vi "Update Generation Signal - Digital.vi"(8 "error in (no error)":errorcluster, 10 "signal update setting":T1, 11 "AudioGeneration in":refnum<class "AudioGeneration.lvclass">) -> (0 "error out":errorcluster, 3 "AudioGeneration out":refnum<class "AudioGeneration.lvclass">)   [LabVIEW 2021, in "AudioGeneration.lvclass"]
uses:
  AudioGeneration.lvclass
  controls/update signal settings.ctl
  <vilib>/NI/STM/TCP/TCP Write Options.ctl
  <vilib>/NI/STM/TCP/Write Message (TCP).vi
  AudioGeneration.lvclass/AudioGeneration.ctl
  <vilib>/NI/STM/NI STM.lvlib
  controls/AudioGenTypeDefs.lvlib
panel:
  out "timeout":bool
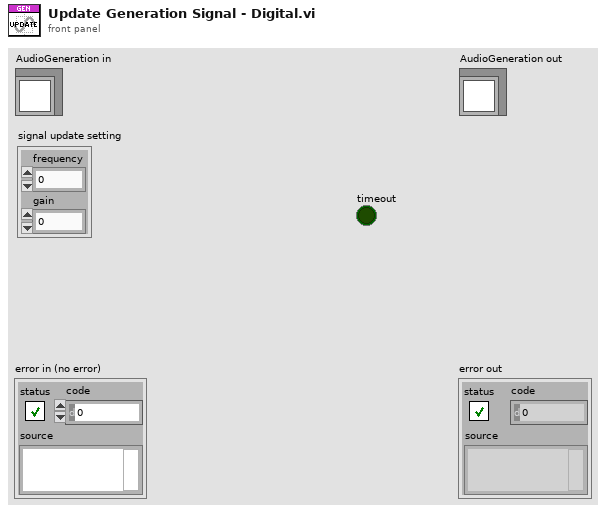
[diagram p1: front panel]
types:
  T1 = typedef "AudioGenTypeDefs.lvlib/update signal settings.ctl" = cluster{"frequency":dbl, "gain":dbl}
  T2 = typedef "NI STM.lvlib/TCP Write Options.ctl" = cluster{"ignore timeout error":bool, "timeout ms (1000)":i32}
  T3 = typedef "NI STM.lvlib/TCP Connection Info.ctl" = cluster{"connection ID":refnum<k5>, "meta data":T4[]}
  T4 = typedef "NI STM.lvlib/MetaDataElement.ctl" = string
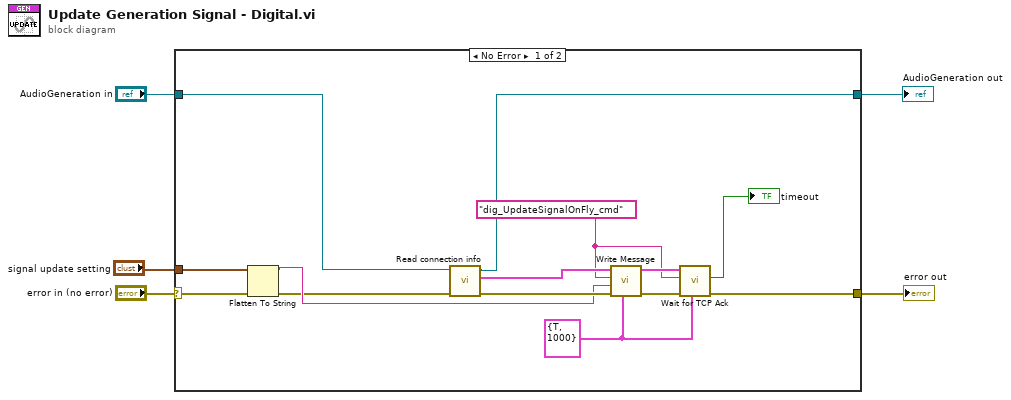
[diagram p0: block diagram]
diagram:
  n1 = case shown="No Error" "error in (no error)" {
    selector: "error in (no error)" -> [w14 w21]
    tunnel: [w16 w21] -> w3
    tunnel: "AudioGeneration in" -> [w7 w20]
    tunnel: [w15 w20] -> w2
    tunnel: "signal update setting" -> [w12 _]
    frame No Error {
      w9 = "dig_UpdateSignalOnFly_cmd" ("name")
      w10 = T2 {"ignore timeout error"=TRUE, "timeout ms (1000)"=1000} ("options")
      n2 = Flatten To String(anything=w12, error in (no error)=w14) -> (data string=w13:string, error out=w6:errorcluster)  [unwired: 2 in, 1 out]
      n3 = call-dynamic "Read connection info.vi"("error in (no error)"=w6, "AudioGeneration in"=w7) -> ("error out"=w18:errorcluster, "connection info"=w19:T3, "AudioGeneration out"=w15:refnum<class "AudioGeneration.lvclass">)  [unwired: 7 in]
      n4 = call-poly <vilib>:"Write Message.vi"("options"=w10, "error in"=w18, "data"=w13, "name"=w9, "connection info in"=w19) -> ("error out"=w17:errorcluster, "connection info out"=w11:T3)  [unwired: 5 in]
      n5 = call "Wait for TCP Ack.vi"("options"=w10, "error in (no error)"=w17, "cmd name"=w9, "connection info in"=w11) -> ("error out"=w16:errorcluster, "timeout"=→"timeout":bool)  [unwired: 4 in, 2 out]
    }
    frame Error {
    }
  }
  "error out" <- w3
  "AudioGeneration out" <- w2
